vi "SM ColorDialog.vi"(8 "错误输入（无错误）":errorcluster, 11 "FullOpen":bool) -> (0 "错误输出":errorcluster, 1 "ShowDialog":i32(ring) items=["None", "OK", "Cancel", "Abort", "Retry", "Ignore", "Yes", "No"], 3 "Color":u32(colorbox) caption="颜色")   [LabVIEW 2012]
uses:
  System.Windows.Forms
  System.Drawing
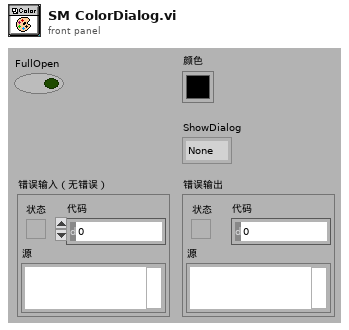
[diagram p1: front panel]
types:
  T1 = enum16{"Constructor", "FullOpen", "ShowDialog", "Get Color", "Dispose", "Close"}
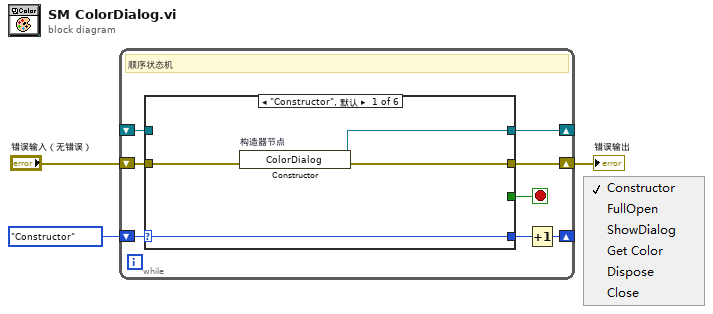
[diagram p0: block diagram]
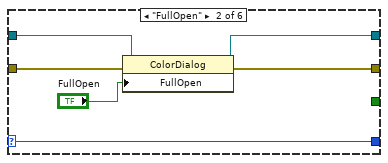
[diagram p2: hidden frame]
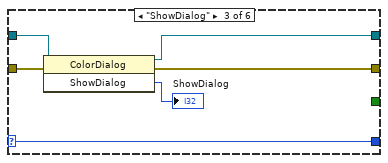
[diagram p3: hidden frame]
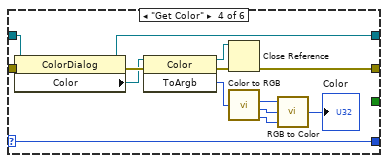
[diagram p4: hidden frame]
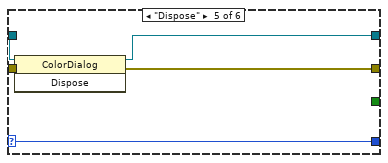
[diagram p5: hidden frame]
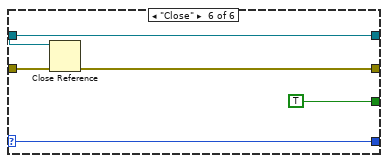
[diagram p6: hidden frame]
diagram:
  n1 = while {
    shift-right: [w9] -> _
    shift-left: T1."Constructor" -> [w11]
    shift-right: [w6] -> w1
    shift-left: "错误输入（无错误）" -> [w8]
    shift-right: [w7] -> _
    shift-left: _ -> [w5]
    stop <- w4 stop-if-true
    # "顺序状态机"
    n2 = case shown="\"Constructor\", 默认" w11 {
      selector: w11 -> [w14 w21 w22 w28 w43 w48]
      tunnel: [w14 w21 w22 w28 w43 w48] -> w10
      tunnel: w8 -> [w15 w19 w26 w40 w45 w51]
      tunnel: [w13 w18 w23 w30 w44 w47] -> w7
      tunnel: [w12 w17 w25 w29 w42 w50] -> w6
      tunnel: w5 -> [_ w20 w27 w41 w46 w47]
      tunnel: [_ _ _ _ _ TRUE] -> w4
      frame "Constructor", Default {
        n3 = constructor on="构造器节点" class="ColorDialog"(error in=w15) -> (reference out=w13:refnum<k24>, error out=w12:errorcluster)  [unwired: 2 in, 1 out]
      }
      frame "FullOpen" {
        n4 = property class="ColorDialog"(reference=w20, error in=w19, "FullOpen"="FullOpen") -> (reference out=w18:refnum<k24>, error out=w17:errorcluster)
      }
      frame "ShowDialog" {
        n5 = invoke class="ColorDialog" method="ShowDialog"(reference=w27, error in=w26) -> (reference out=w23:refnum<k24>, error out=w25:errorcluster, "ShowDialog"=→"ShowDialog":i32)  [unwired: 1 in]
      }
      frame "Get Color" {
        n6 = property class="ColorDialog"(reference=w41, error in=w40) -> (reference out=w30:refnum<k24>, error out=w39:errorcluster, "Color"=w38:refnum<k24>)
        n7 = invoke class="Color" method="ToArgb"(reference=w38, error in=w39) -> (reference out=w31:refnum<k24>, error out=w32:errorcluster, "ToArgb"=w33:i32)  [unwired: 1 in]
        n8 = Close Reference(reference=w31, error in (no error)=w32) -> (error out=w29:errorcluster)
        n9 = call <vilib>:"Color to RGB.vi"("Color"=w33) -> ("R"=w34:u8, "G"=w35:u8, "B"=w36:u8)  [unwired: 1 out]
        n10 = call <vilib>:"RGB to Color.vi"("B"=w36, "G"=w35, "R"=w34) -> ("Color"=→"Color":u32)
      }
      frame "Dispose" {
        n11 = invoke class="ColorDialog" method="Dispose"(reference=w46, error in=w45) -> (reference out=w44:refnum<k24>, error out=w42:errorcluster)  [unwired: 1 in, 1 out]
      }
      frame "Close" {
        n12 = Close Reference(reference=w47, error in (no error)=w51) -> (error out=w50:errorcluster)
      }
    }
    n13 = Increment(x=w10) -> (x+1=w9:T1)
  }
  "错误输出" <- w1
